vi "Calibrate ITEMP.vi"(8 "error in (no error)":errorcluster, 9 "Position in":u32, 10 "Cree Comms in":refnum<class "Cree Communications.lvclass">, 11 "Calibration in":refnum<class "Calibration.lvclass">) -> (0 "error out":errorcluster, 1 "Position out":u32, 2 "Cree Comms out":refnum<class "Cree Communications.lvclass">, 3 "Calibration out":refnum<class "Calibration.lvclass">, 4 "Passed":bool, 6 "Fail Code":string)   [LabVIEW 2015, in "Calibration.lvclass"]
uses:
  Calibration.lvclass
  Classes/Cree Communications/Class/Cree Communications.lvclass
  Classes/Application/Class/Application.lvclass
  Test Class/Test Class.lvclass
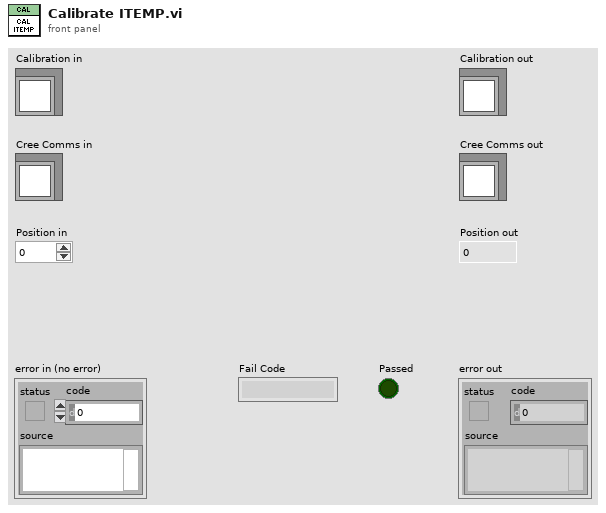
[diagram p1: front panel]
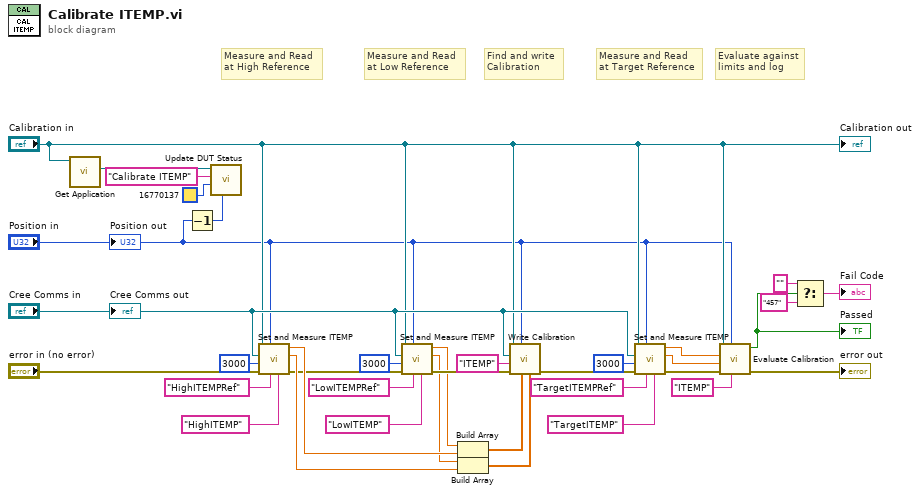
[diagram p0: block diagram]
diagram:
  # "Evaluate against\nlimits and log"
  # "Measure and Read\nat Target Reference"
  # "Find and write\nCalibration"
  # "Measure and Read\nat Low Reference"
  # "Measure and Read\nat High Reference"
  n1 = call "Get Application.vi"("Test Class in"="Calibration in") -> ("Application.lvlib:Application.lvclass"=w3:refnum<class "Application.lvclass">)  [unwired: 9 in, 1 out]
  n2 = Decrement(x="Position in") -> (x-1=w2:u32)
  n3 = call "Update DUT Status.vi"("Position"=w2, "BG Color"=u32 16770137, "Message ('')"="Calibrate ITEMP", "Application in"=w3) -> ()  [unwired: 6 in, 2 out]
  n4 = call "Set and Measure ITEMP.vi"("Header"="HighITEMP" ("Name"), "Name"="HighITEMPRef", "Position in"="Position in", "error in (no error)"="error in (no error)", "Measurement Wait Time"=u32 3000, "Cree Comms in"="Cree Comms in", "Calibration in"="Calibration in") -> ("error out"=w21:errorcluster, "DSpic Measurement"=w26:dbl, "Actual Measurement"=w25:dbl)  [unwired: 2 in]
  n5 = call "Set and Measure ITEMP.vi"("Header"="LowITEMP" ("Name"), "Name"="LowITEMPRef", "Position in"="Position in", "error in (no error)"=w21, "Measurement Wait Time"=u32 3000, "Cree Comms in"="Cree Comms in", "Calibration in"="Calibration in") -> ("error out"=w18:errorcluster, "DSpic Measurement"=w17:dbl, "Actual Measurement"=w16:dbl)  [unwired: 2 in]
  n6 = Build Array(w16, w25) -> (w35:dbl[])
  n7 = Build Array(w17, w26) -> (w36:dbl[])
  n8 = call "Write Calibration.vi"("DSPic Measurements"=w36, "Actual Measurements"=w35, "Position in"="Position in", "error in (no error)"=w18, "Calibration Type"="ITEMP", "Cree Comms in"="Cree Comms in", "Calibration in"="Calibration in") -> ("error out"=w14:errorcluster)  [unwired: 4 in]
  n9 = call "Set and Measure ITEMP.vi"("Header"="TargetITEMP" ("Name"), "Name"="TargetITEMPRef", "Position in"="Position in", "error in (no error)"=w14, "Measurement Wait Time"=u32 3000, "Cree Comms in"="Cree Comms in", "Calibration in"="Calibration in") -> ("error out"=w9:errorcluster, "DSpic Measurement"=w10:dbl, "Actual Measurement"=w11:dbl)  [unwired: 2 in]
  n10 = call "Evaluate Calibration.vi"("Calibration Type"="ITEMP" ("Name"), "Position"="Position in", "Error in"=w9, "DSPic Measurement"=w10, "Actual Measurement"=w11, "Calibration in"="Calibration in") -> ("Error out"=→"error out":errorcluster, "Passed"=w30:bool)  [unwired: 4 in]
  "Passed" <- w30
  n11 = Select(t="", s=w30, f="457") -> (s? t:f=→"Fail Code":string)
  "Calibration out" <- "Calibration in"
  "Position out" <- "Position in"
  "Cree Comms out" <- "Cree Comms in"
